vi "Run Test Case.vi"(8 "error in (no error)":errorcluster, 10 "Test Case":refnum<class "LUnit Test Case.lvclass">, 11 "Execution API In":refnum<class "Execution API.lvclass">) -> (0 "error out":errorcluster, 3 "Execution API Out":refnum<class "Execution API.lvclass">)   [LabVIEW 2020, in "Execution API.lvclass"]
doc: "Run a single test case."
uses:
  Execution API.lvclass
  C:/Users/anton/Documents/GitHub/LUnit/source/Application Framework/Process Classes/Process/Process.lvclass
  Test Case/LUnit Test Case.lvclass
  Application Framework/Process Classes/Process/Process.lvclass/Process.ctl
  Application Framework/Process Classes/Process/Process.lvclass
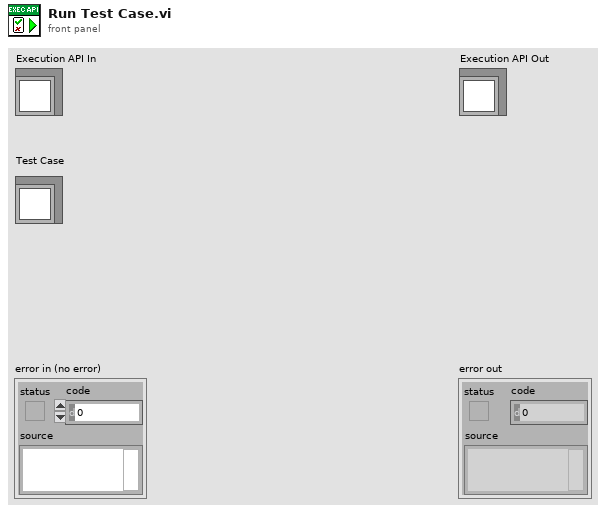
[diagram p1: front panel]
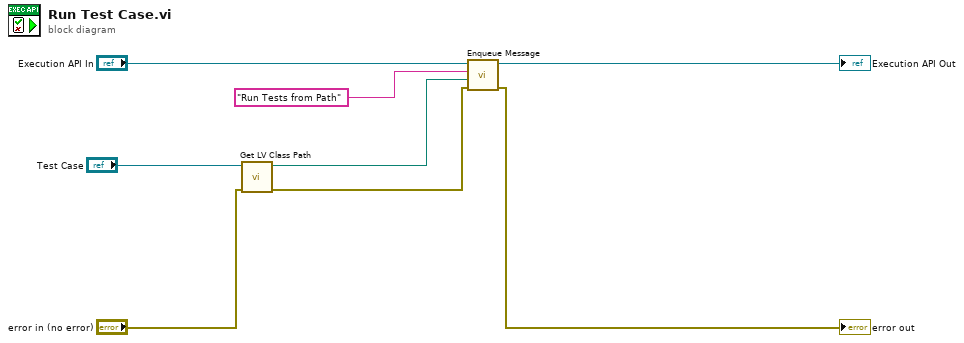
[diagram p0: block diagram]
diagram:
  n1 = call <vilib>:"Get LV Class Path.vi"("error in (no error)"="error in (no error)", "object"="Test Case") -> ("error out"=w1:errorcluster, "class path"=w3:path)  [unwired: 8 in]
  n2 = call "Enqueue Message.vi"("error in (no error)"=w1, "Message Data"=w3, "Message"="Run Tests from Path", "Process In"="Execution API In") -> ("error out"=→"error out":errorcluster, "Process Out"=→"Execution API Out":refnum<class "Execution API.lvclass">)  [unwired: 6 in]
